vi "Append Paragraph with Link [ ].vi"(0 "PDF Report":refnum<class "PDF Report Class.lvclass">, 2 "Text [ ]":T3, 11 "error in (no error)":errorcluster, 13 "Image to Add [ ]":T1 {"Scale" format="%#_g %"}) -> (4 "PDF Report duplicate":refnum<class "PDF Report Class.lvclass">, 15 "error out":errorcluster)   [LabVIEW 2019]
doc: "<B>Only ASCII or UTF-16 (no-bidi).</B>\n\nAppends text with a <B>line feed</B>, at the end, to the PDF report. This text can be <B>aligned</B> (CENTER, JUSTIFY, LEFT, RIGHT) and <B>indented</B>. \n\nIf <B>Font</B> and <B>Pararaph properties</B> are not specified then the <B>Default font</B> and <B>Default paragraph</B> will be use.\n\nThe data type you wire to the <B>Text</B> input determines the polymorphic instance to use.\n\n<B>FRANÇAIS</B>\nAjoute au rapport PDF du texte sous la forme d'un paragraphe terminé avec un \"<B>Line Feed</B>\". Ce texte peut être <B>aligné</B> (CENTER, JUSTIFY, LEFT, RIGHT) et avoir un <B>renfoncement</B> (gauche et droit) pour tout le paragraphe.\n\nSi la police de caractères <B>Font</B> et les propriétés <B>Pararaph properties</B> ne sont pas spécifiés alors la police par défaut <B>Default font</B> et <B>Default paragraph</B> seront utilisées.\n\nLe type de données que vous connectez au terminal <B>Text</B> détermine l'instance polymorphique utilisée.\n\nVersion 2.0\nDeveloped by Jean-Marc Simard\nCopyright © 2012, Exaprom Inc.\nAll rights reserved.\nLicense: BSD\n\nWith iTextSharp 4.1.6 (http://itextsharp.sourceforge.net)\nunder Mozilla Public License Version 1.1\n(http://www.mozilla.org/MPL/MPL-1.1.html)"
uses:
  <userlib>/Exaprom PDF/LV Class/PDF Report Class/PDF Report Class.lvclass
  <userlib>/Exaprom PDF/Controls/Text Controls/Text and hyperlink [ ].ctl
  <userlib>/Exaprom PDF/Controls/Text Controls/Text from String of File and hyperlink.ctl
  <userlib>/Exaprom PDF/Controls/Font Controls/Font complete cluster horizontal.ctl
  <userlib>/Exaprom PDF/Controls/Font Controls/Font size.ctl
  <userlib>/Exaprom PDF/Controls/Font Controls/Font color.ctl
  <userlib>/Exaprom PDF/Controls/Font Controls/Type and encoding.ctl
  <userlib>/Exaprom PDF/Controls/Text Controls/Unicode/Type and run direction.ctl
  <userlib>/Exaprom PDF/Controls/Initialization Controls/Defaut Paragraphe and Line Spacing.ctl
  <userlib>/Exaprom PDF/Controls/Text Controls/Texte alignement.ctl
  <userlib>/Exaprom PDF/Controls/Text Controls/Line spacing.ctl
  <userlib>/Exaprom PDF/Controls/Text Controls/Paragraph indentation.ctl
  <userlib>/Exaprom PDF/Controls/General Controls/Image to Add [ ].ctl
  <userlib>/Exaprom PDF/Controls/Image Controls/Image Scale.ctl
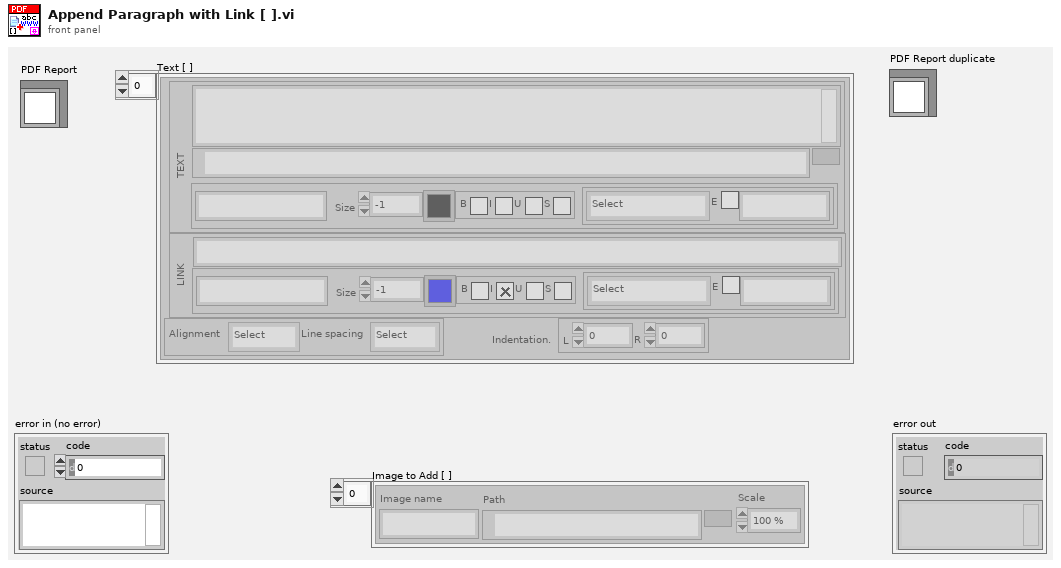
[diagram p1: front panel]
types:
  T1 = typedef "Image to Add [ ].ctl" = cluster{"Image name":string, "Path":path, "Scale":T2}[]
  T2 = typedef "Image Scale.ctl" = sgl
  T3 = typedef "Text and hyperlink [ ].ctl" = T4[]
  T4 = typedef "Text from String of File and hyperlink.ctl" = cluster{"Text":cluster{"Text":string, "Path":path, "Font complete":T5}, "Link":cluster{"Hyperlink":string, "Font complete":T5}, "Paragraphe":T10, "Indentation":T13}
  T5 = typedef "Font complete cluster horizontal.ctl" = cluster{"Name":string, "Size":T6, "Color":T7, "Style":cluster{"Bold":bool, "Italic":bool, "Underline":bool, "Strikeout":bool}, "Type":T8}
  T6 = typedef "Font size.ctl" = sgl
  T7 = typedef "Font color.ctl" = u32
  T8 = typedef "Type and encoding.ctl" = cluster{"Type&direction":T9, "Embedded":bool, "Encoding":string}
  T9 = typedef "Type and run direction.ctl" = enum16{"Select", "ASCII", "UTF-16", "UTF-16 (default)", "UTF-16 (LTR)", "UTF-16 (RTL)"}
  T10 = typedef "Defaut Paragraphe and Line Spacing.ctl" = cluster{" Aligment":T11, "Line spacing":T12}
  T11 = typedef "Texte alignement.ctl" = enum16{"Select", "CENTER", "JUSTIFY", "LEFT", "RIGHT"}
  T12 = typedef "Line spacing.ctl" = enum16{"Select", "1.0", "1.5", "2.0"}
  T13 = typedef "Paragraph indentation.ctl" = cluster{"Left":sgl, "Right":sgl}
  T14 = typedef "Image to Add refnum [ ].ctl" = cluster{"Image name":string, "InstanceImage":refnum<k24>}[]
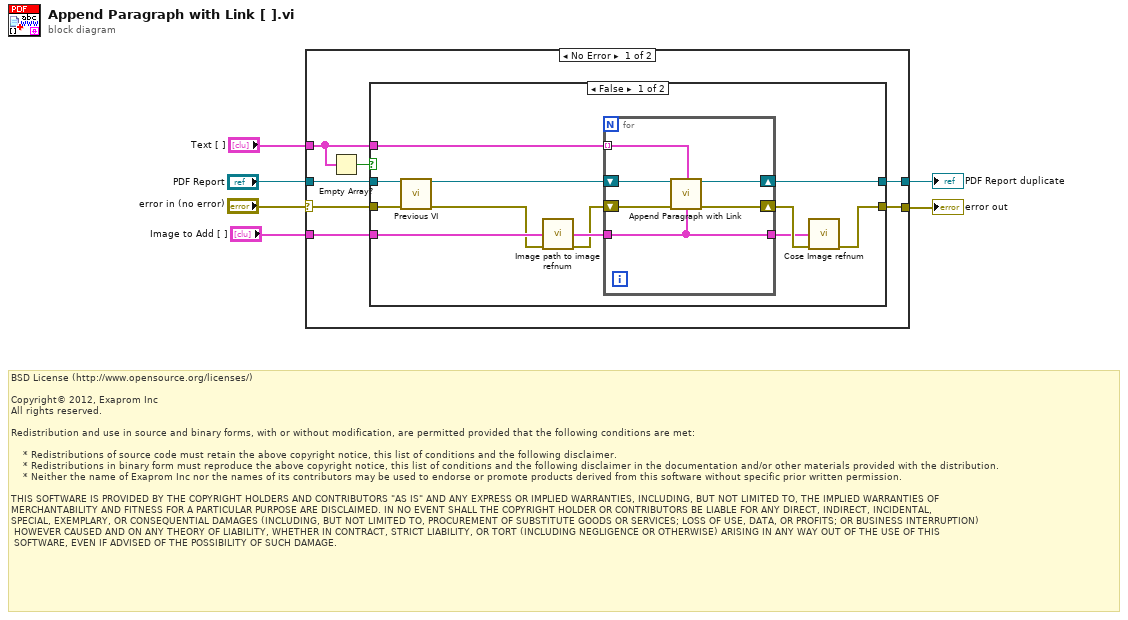
[diagram p0: block diagram]
diagram:
  # "BSD License (http://www.opensource.org/licenses/)\n\nCopyright© 2012, Exaprom Inc\nAll rights reserved.\n\nRedistribution and use in source and binary forms, with or without modification, are permitted provided that the following conditions are met:\n\n    * Redistributions of source code must retain the above copyright notice, this list of conditions and the following disclaimer.\n    * Redistributions in binary form must reproduce the above copyright notice, this list of conditions and the following disclaimer in the documentation and/or other materials provided with the distribution.\n    * Neither the name of Exaprom Inc nor the names of its contributors may be used to endorse or promote products derived from this software without specific prior written permission.\n\nTHIS SOFTWARE IS PROVIDED BY THE COPYRIGHT HOLDERS AND CONTRIBUTORS \"AS IS\" AND ANY EXPRESS OR IMPLIED WARRANTIES, INCLUDING, BUT NOT LIMITED TO, THE IMPLIED WARRANTIES OF \nMERCHANTABILITY AND FITNESS FOR A PARTICULAR PURPOSE ARE DISCLAIMED. IN NO EVENT SHALL THE COPYRIGHT HOLDER OR CONTRIBUTORS BE LIABLE FOR ANY DIRECT, INDIRECT, INCIDENTAL,\nSPECIAL, EXEMPLARY, OR CONSEQUENTIAL DAMAGES (INCLUDING, BUT NOT LIMITED TO, PROCUREMENT OF SUBSTITUTE GOODS OR SERVICES; LOSS OF USE, DATA, OR PROFITS; OR BUSINESS INTERRUPTION)\n HOWEVER CAUSED AND ON ANY THEORY OF LIABILITY, WHETHER IN CONTRACT, STRICT LIABILITY, OR TORT (INCLUDING NEGLIGENCE OR OTHERWISE) ARISING IN ANY WAY OUT OF THE USE OF THIS\n SOFTWARE, EVEN IF ADVISED OF THE POSSIBILITY OF SUCH DAMAGE."
  n1 = case shown="No Error" "error in (no error)" {
    selector: "error in (no error)" -> [w12 w35]
    tunnel: [w10 w35] -> w6
    tunnel: "PDF Report" -> [w11 w34]
    tunnel: [w13 w34] -> w3
    tunnel: "Text [ ]" -> [w9 _]
    tunnel: "Image to Add [ ]" -> [w7 _]
    frame No Error {
      n2 = Empty Array?(array=w9) -> (empty?=w8:bool)
      n3 = case shown="False" w8 {
        tunnel: [w23 w33] -> w13
        tunnel: w12 -> [w16 w32]
        tunnel: w11 -> [w24 w33]
        tunnel: [w18 w32] -> w10
        tunnel: w9 -> [w25 _]
        tunnel: w7 -> [w22 _]
        frame False {
          n4 = call <userlib>:"Previous VI.vi"("PDF Report IN"=w24, "error in (no error)"=w16) -> ("PDF Report OUT"=w15:refnum<class "PDF Report Class.lvclass">, "error out"=w14:errorcluster)  [unwired: 12 out]
          n5 = call <userlib>:"Image path to image refnum.vi"("Image to Add [ ]"=w22, "error in (no error)"=w14) -> ("Image to Add refnum [ ]"=w21:T14, "error out"=w20:errorcluster)  [unwired: 12 out]
          n6 = for {
            shift-right: [w29] -> w19
            shift-left: w20 -> [w30]
            shift-right: [w31] -> w23
            shift-left: w15 -> [w28]
            tunnel: w25 -> [w27] mode=indexing
            tunnel: w21 -> [w26]
            tunnel: [w26] -> w17
            n7 = call <userlib>:"Append Paragraph with Link.vi"("PDF Report"=w28, "Text"=w27, "error in (no error)"=w30, "Image to Add refnum [ ]"=w26) -> ("PDF Report duplicate"=w31:refnum<class "PDF Report Class.lvclass">, "error out"=w29:errorcluster)  [unwired: 10 out]
          }
          n8 = call <userlib>:"Cose Image refnum.vi"("Image to Add refnum [ ]"=w17, "error in (no error)"=w19) -> ("error out"=w18:errorcluster)  [unwired: 13 out]
        }
        frame True {
        }
      }
    }
    frame Error {
    }
  }
  "error out" <- w6
  "PDF Report duplicate" <- w3
